vi "Roiausposition.vi"(11 "Cluster":cluster{dbl, dbl, dbl, dbl}) -> (2 "ROI Descriptor":T1 {"Contours"."Type" items=["No Selection", "Point", "Line", "Rectangle", "Oval", "Polygon", "Freehand Region", "Annulus", "Unused2", "Unused3", "Broken Line", "Freehand Line", "Rotated Rectangle"]}, 3 "Boolean":bool)   [LabVIEW 2014]
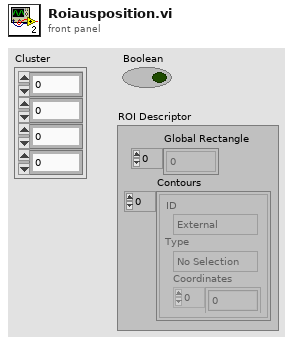
[diagram p1: front panel]
types:
  T1 = typedef "ROI Descriptor" = cluster{"Global Rectangle":i32[], "Contours":cluster{"ID":enum32{"External", "Internal"}, "Type":u32, "Coordinates":i32[]}[]}
  T2 = typedef "IMAQ Rectangle" = cluster{"Left":i32, "Top":i32, "Right":i32, "Bottom":i32, "Rotation":dbl}
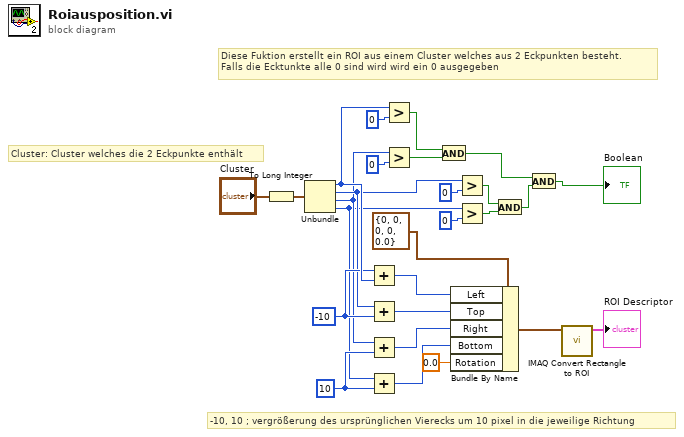
[diagram p0: block diagram]
diagram:
  w13 = 10 ("y")
  w14 = -10 ("x")
  # "-10, 10 ; vergrößerung des ursprünglichen Vierecks um 10 pixel in die jeweilige Richtung"
  # "Cluster: Cluster welches die 2 Eckpunkte enthält"
  # "Diese Fuktion erstellt ein ROI aus einem Cluster welches aus 2 Eckpunkten besteht. \nFalls die Ecktunkte alle 0 sind wird wird ein 0 ausgegeben"
  n1 = To Long Integer(number="Cluster") -> (32bit integer=w17:cluster{i32, i32, i32, i32})
  n2 = Unbundle(w17) -> (w15:i32, w8:i32, w7:i32, w6:i32)
  n3 = Add(x=w14, y=w15) -> (x+y=w12:i32)
  n4 = Add(x=w8, y=w14) -> (x+y=w11:i32)
  n5 = Add(x=w7, y=w13) -> (x+y=w10:i32)
  n6 = Add(x=w6, y=w13) -> (x+y=w9:i32)
  n7 = Greater?(x=w15, y=0) -> (0:w25:bool)
  n8 = Greater?(x=w7, y=0) -> (0:w27:bool)
  n9 = And(x=w25, y=w27) -> (x .and. y?=w26:bool)
  n10 = Bundle By Name(cluster=T2 {"Left"=0, "Top"=0, "Right"=0, "Bottom"=0, "Rotation"=0.0} ("Rectangle"), "Left"=w12, "Top"=w11, "Right"=w10, "Bottom"=w9, "Rotation"=0.0) -> (w20:T2)
  n11 = Greater?(x=w8, y=0) -> (0:w4:bool)
  n12 = Greater?(x=w6, y=0) -> (0:w3:bool)
  n13 = And(x=w4, y=w3) -> (x .and. y?=w1:bool)
  n14 = And(x=w26, y=w1) -> (x .and. y?=→"Boolean":bool)
  n15 = call "IMAQ Convert Rectangle to ROI"("Rectangle"=w20) -> ("ROI Descriptor"=→"ROI Descriptor":T1)  [unwired: 8 in, 1 out]
